vi "CAN Read FD.vi"(8 "error in (no error)":errorcluster, 9 "TimestampBuffer":T2, 10 "MessageBuffer":T1, 11 "Channel":u16) -> (0 "error out":errorcluster, 1 "TimestampBuffer out":T2, 2 "MessageBuffer out":T1, 3 "function return":u32)   [LabVIEW 2020, in "PCANBasic.lvlib"]
doc: "TPCANStatus __stdcall CAN_Read(\n TPCANHandle Channel, \n TPCANMsg* MessageBuffer, \n TPCANTimestamp* TimestampBuffer);"
uses:
  PCANBasic.lvlib
  <userlib>/PCANBasic/PCANBasic.dll
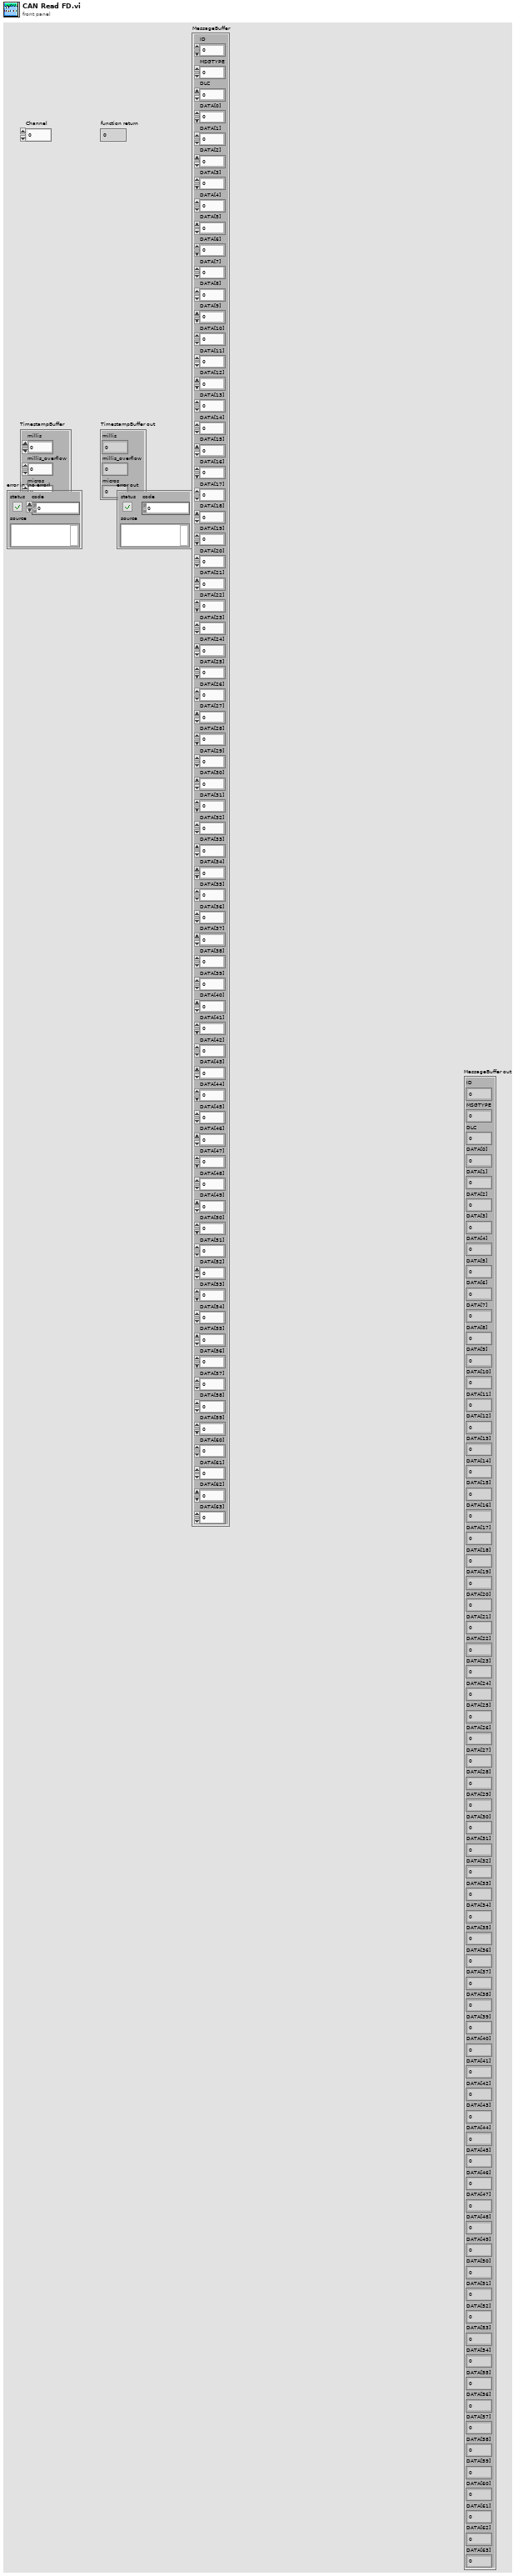
[diagram p1: front panel]
types:
  T1 = cluster{"ID":u32, "MSGTYPE":u8, "DLC":u8, "DATA[0]":u8, "DATA[1]":u8, "DATA[2]":u8, "DATA[3]":u8, "DATA[4]":u8, "DATA[5]":u8, "DATA[6]":u8, "DATA[7]":u8, "DATA[8]":u8, "DATA[9]":u8, "DATA[10]":u8, "DATA[11]":u8, "DATA[12]":u8, "DATA[13]":u8, "DATA[14]":u8, "DATA[15]":u8, "DATA[16]":u8, "DATA[17]":u8, "DATA[18]":u8, "DATA[19]":u8, "DATA[20]":u8, "DATA[21]":u8, "DATA[22]":u8, "DATA[23]":u8, "DATA[24]":u8, "DATA[25]":u8, "DATA[26]":u8, "DATA[27]":u8, "DATA[28]":u8, "DATA[29]":u8, "DATA[30]":u8, "DATA[31]":u8, "DATA[32]":u8, "DATA[33]":u8, "DATA[34]":u8, "DATA[35]":u8, "DATA[36]":u8, "DATA[37]":u8, "DATA[38]":u8, "DATA[39]":u8, "DATA[40]":u8, "DATA[41]":u8, "DATA[42]":u8, "DATA[43]":u8, "DATA[44]":u8, "DATA[45]":u8, "DATA[46]":u8, "DATA[47]":u8, "DATA[48]":u8, "DATA[49]":u8, "DATA[50]":u8, "DATA[51]":u8, "DATA[52]":u8, "DATA[53]":u8, "DATA[54]":u8, "DATA[55]":u8, "DATA[56]":u8, "DATA[57]":u8, "DATA[58]":u8, "DATA[59]":u8, "DATA[60]":u8, "DATA[61]":u8, "DATA[62]":u8, "DATA[63]":u8}
  T2 = cluster{"millis":u32, "millis_overflow":u16, "micros":u16}
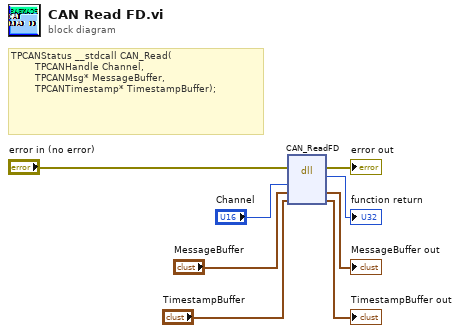
[diagram p0: block diagram]
diagram:
  # "TPCANStatus __stdcall CAN_Read(\n        TPCANHandle Channel, \n        TPCANMsg* MessageBuffer, \n        TPCANTimestamp* TimestampBuffer);"
  n1 = dll-call lib="D:/Program Files (x86)/National Instruments/LabVIEW 2020/user.lib/PCANBasic/PCANBasic.*" fn="CAN_ReadFD"(error in="error in (no error)", "Channel"="Channel", "MessageBuffer out"="MessageBuffer", "TimestampBuffer"="TimestampBuffer") -> (error out=→"error out":errorcluster, "返回类型"=→"function return":u32, "MessageBuffer out"=→"MessageBuffer out":T1, "TimestampBuffer"=→"TimestampBuffer out":T2)  [unwired: 3 in, 1 out]
